vi "Assert Not Equal Value and Type_Variant.vi"(4 "Execution time (s)":dbl=-1.0, 6 "error code (1)":i32=1, 7 "Label":string, 8 "error in":errorcluster, 10 "Y":variant, 11 "X":variant) -> (0 "error out":errorcluster, 2 "Properties":refnum<class "Properties.Assert.lvclass">)   [LabVIEW 2021, in "Bananas.lvlib"]
uses:
  Bananas.lvlib
  <vilib>/addons/_JKI Toolkits/Caraya/classes/Properties.Assert/Properties.Assert.lvclass
  Banana/Banana.lvclass/Banana.ctl
  AssertEqualValue/AssertEqualValue.lvclass/AssertEqualValue.ctl
  AssertEqualType/AssertEqualType.lvclass/AssertEqualType.ctl
  AssertEqualType/Write X.vi
  AssertEqualType/Write Y.vi
  AssertEqualType/Write Not_.vi
  AssertEqualValue/Write X.vi
  AssertEqualValue/Write Y.vi
  AssertEqualValue/Write Not_.vi
  AssertEqualType/AssertEqualType.lvclass
  C:/Repositories/LVOS/Bananas/lv-src/Bananas/BananaPeel/BananaPeel.lvclass
  AssertEqualValue/AssertEqualValue.lvclass
  <vilib>/addons/_JKI Toolkits/Caraya/classes/Assert/Assert.lvclass
  Banana/Banana.lvclass
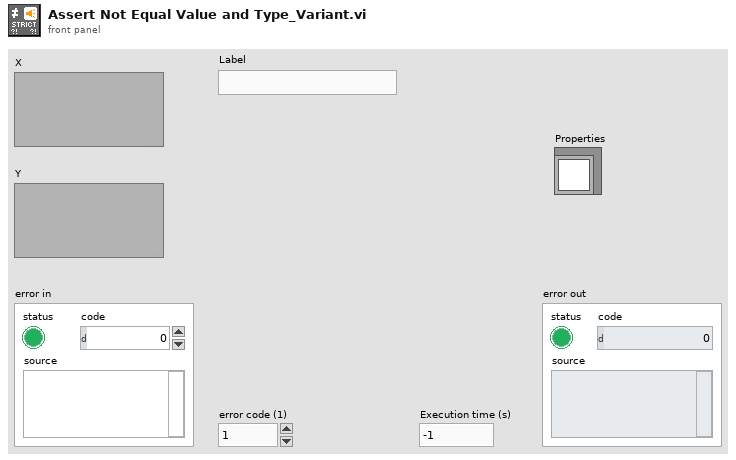
[diagram p1: front panel]
types:
  T1 = typedef "Bananas.lvlib/Assertion Strategies -- cluster.ctl" = cluster{"AssertTrue":refnum<class "AssertTrue.lvclass">, "AssertFalse":refnum<class "AssertFalse.lvclass">, "AssertEqualValue":refnum<class "AssertEqualValue.lvclass">, "AssertEqualType":refnum<class "AssertEqualType.lvclass">, "AssertCompareValue":refnum<class "AssertCompareValue.lvclass">, "AssertError":refnum<class "AssertError.lvclass">, "AssertAlmostEqual":refnum<class "AssertAlmostEqualValue.lvclass">}
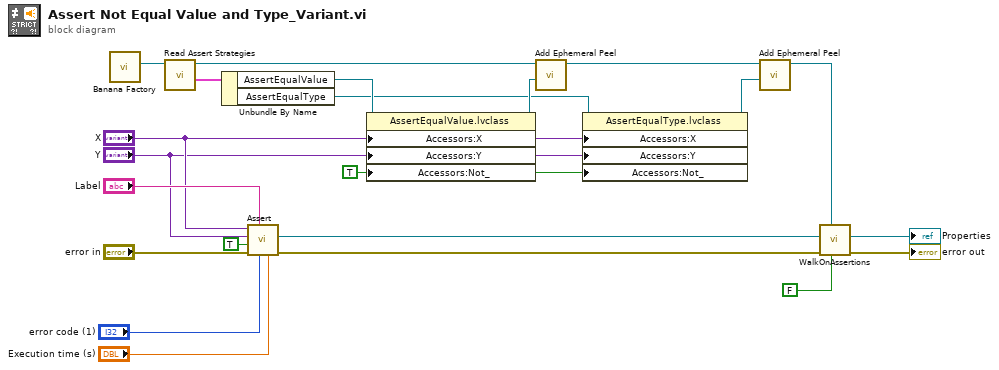
[diagram p0: block diagram]
diagram:
  w5 = TRUE ("Not_")
  n1 = call "Banana Factory.vi"() -> ("Bunch"=w13:refnum<class "Banana.lvclass">)  [unwired: 10 in, 1 out]
  n2 = call "Read Assert Strategies.vi"("Banana in"=w13) -> ("Strategies"=w11:T1, "Banana out"=w12:refnum<class "Banana.lvclass">)  [unwired: 9 in]
  n3 = Unbundle By Name(w11) -> ("AssertEqualValue"=w9:refnum<class "AssertEqualValue.lvclass">, "AssertEqualType"=w7:refnum<class "AssertEqualType.lvclass">)
  n4 = call-poly <vilib>:"Assert.vi"("Execution time (s)"="Execution time (s)", "error code (1)"="error code (1)", "Label"="Label", "error in (no error)"="error in", "Register with caller test (F)"=TRUE, "Y"="Y", "X"="X") -> ("error out"=w17:errorcluster, "Properties.Assert"=w15:refnum<class "Properties.Assert.lvclass">)  [unwired: 3 in]
  n5 = property class="AssertEqualValue.lvclass"(reference=w9, "Accessors:X"="X", "Accessors:Y"="Y", "Accessors:Not_"=w5) -> (reference out=w8:refnum<class "AssertEqualValue.lvclass">)  [unwired: 1 in, 1 out]
  n6 = call "Add Ephemeral Peel.vi"("BananaPeel"=w8, "Bunch"=w12) -> ("Bunch"=w10:refnum<class "Banana.lvclass">)  [unwired: 9 in]
  n7 = property class="AssertEqualType.lvclass"(reference=w7, "Accessors:X"="X", "Accessors:Y"="Y", "Accessors:Not_"=w5) -> (reference out=w6:refnum<class "AssertEqualType.lvclass">)  [unwired: 1 in, 1 out]
  n8 = call "Add Ephemeral Peel.vi"("BananaPeel"=w6, "Bunch"=w10) -> ("Bunch"=w2:refnum<class "Banana.lvclass">)  [unwired: 9 in]
  n9 = call "WalkOnAssertions.vi"("Stop on 1st fail"=FALSE, "Bunch"=w2, "error in (no error)"=w17, "Properties"=w15) -> ("error out"=→"error out":errorcluster, "Properties out"=→"Properties":refnum<class "Properties.Assert.lvclass">)  [unwired: 6 in]
